vi "Standard Error Behavior.vi"() -> ()   [LabVIEW 2017, in "Assertions.Tests.lvlib"]
uses:
  Assertions.Tests.lvlib
  <vilib>/Utility/error.llb/Error Cluster From Error Code.vi
  src/Transparent Assertions/Constraints/IsEqual/Create.vi
  <vilib>/ErrorRing/Error Ring.xnode
  src/Transparent Assertions/Constraints/IsEqual/IsEqual.lvclass
  src/Transparent Assertions/Assertions/Assertions.lvlib
panel:
  out "error out":errorcluster
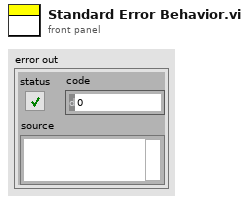
[diagram p1: front panel]
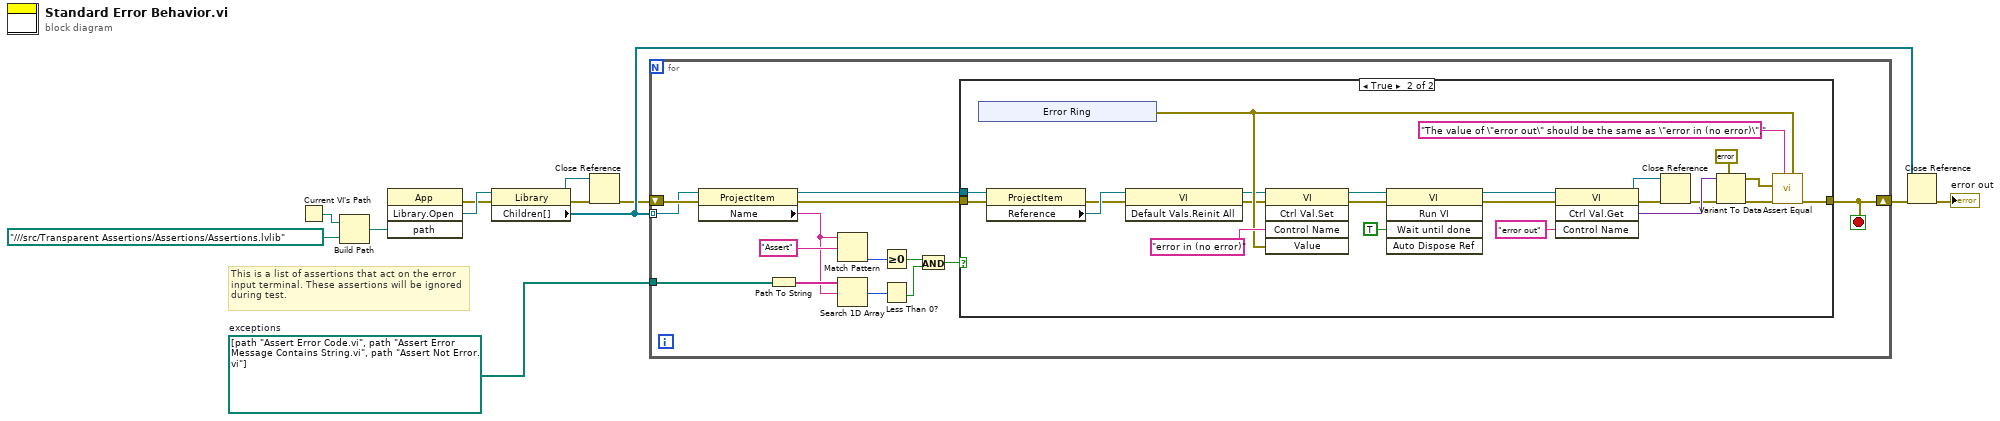
[diagram p0: block diagram]
diagram:
  w5 = path[] [path "Assert Error Code.vi", path "Assert Error Message Contains String.vi", path "Assert Not Error.vi"]  # exceptions
  # "This is a list of assertions that act on the error\ninput terminal. These assertions will be ignored\nduring test."
  n1 = Current VI's Path() -> (path=w11:path)
  n2 = Build Path(base path=w11, name or relative path=path "../../../src/Transparent Assertions/Assertions/Assertions.lvlib") -> (appended path=w9:path)
  n3 = invoke class="App" method="Library.Open"("path"=w9) -> (error out=w7:errorcluster, "Open Library"=w8:refnum<vi>)  [unwired: 3 in, 2 out]
  n4 = property class="Library"(reference=w8, error in=w7) -> (reference out=w1:refnum<vi>, error out=w6:errorcluster, "Children[]"=w3:refnum<vi>[])
  n5 = Close Reference(reference=w1, error in (no error)=w6) -> (error out=w2:errorcluster)
  n6 = for {
    tunnel: w3 -> [w25] mode=indexing
    tunnel: w5 -> [w20]
    shift-right: [w21] -> w12
    shift-left: w2 -> [w26]
    stop <- w21 stop-if-true
    n7 = property class="ProjectItem"(reference=w25, error in=w26) -> (reference out=w23:refnum<vi>, error out=w22:errorcluster, "Name"=w18:string)
    n8 = Path To String(path=w20) -> (string=w19:string[])
    n9 = Match Pattern(string=w18, regular expression="Assert") -> (offset past match=w17:i32)  [unwired: 1 in, 3 out]
    n10 = Search 1D Array(1D array=w19, element=w18) -> (index of element=w15:i32)  [unwired: 1 in]
    n11 = Greater Or Equal To 0?(x=w17) -> (x >= 0?=w16:bool)
    n12 = Less Than 0?(x=w15) -> (x < 0?=w14:bool)
    n13 = And(x=w16, y=w14) -> (x .and. y?=w13:bool)
    n14 = case shown="True" w13 {
      tunnel: w23 -> [_ w36]
      tunnel: w22 -> [w27 w35]
      tunnel: [w27 w42] -> w21
      frame False {
      }
      frame True {
        n15 = xnode "Error Ring"() -> ("error out"=w41:errorcluster)
        n16 = property class="ProjectItem"(reference=w36, error in=w35) -> (error out=w30:errorcluster, "Reference"=w31:refnum<vi>)  [unwired: 1 out]
        n17 = invoke class="VI" method="Default Vals.Reinit All"(reference=w31, error in=w30) -> (reference out=w32:refnum<vi>, error out=w33:errorcluster)  [unwired: 1 in, 1 out]
        n18 = invoke class="VI" method="Ctrl Val.Set"(reference=w32, error in=w33, "Control Name"="error in (no error)", "Value"=w41) -> (reference out=w48:refnum<vi>, error out=w49:errorcluster)  [unwired: 1 in, 3 out]
        n19 = invoke class="VI" method="Run VI"(reference=w48, error in=w49, "Wait until done"=TRUE ("Wait Until Done")) -> (reference out=w45:refnum<vi>, error out=w46:errorcluster)  [unwired: 2 in, 3 out]
        n20 = invoke class="VI" method="Ctrl Val.Get"(reference=w45, error in=w46, "Control Name"="error out") -> (reference out=w28:refnum<vi>, error out=w43:errorcluster, "Get Control Value Variant"=w39:variant)  [unwired: 1 in, 1 out]
        n21 = Close Reference(reference=w28, error in (no error)=w43) -> (error out=w29:errorcluster)
        n22 = Variant To Data(error in=w29, type=errorcluster {"status"=FALSE, "code"=0, "source"=""} ("error constant"), Variant=w39) -> (data=w37:errorcluster, error out=w40:errorcluster)
        n23 = call "Assert Equal.vi"("Expected"=w41, "Message (\"\")"="The value of \"error out\" should be the same as \"error in (no error)\"." ("Message (\"\")"), "error in (no error)"=w40, "Actual"=w37) -> ("error out"=w42:errorcluster)  [unwired: 7 in]
      }
    }
  }
  n24 = Close Reference(reference=w3, error in (no error)=w12) -> (error out=→"error out":errorcluster)
